vi "Write Signal Generator.lvclass.vi"(10 "Signal Generator.lvclass":refnum<class "Signal Generator.lvclass">, 11 "Harmonics in":refnum<class "Harmonics.lvclass">) -> (3 "Harmonics out":refnum<class "Harmonics.lvclass">)   [LabVIEW 2020, in "Harmonics.lvclass"]
uses:
  Harmonics.lvclass
  Instruments/Signal Generator/Signal Generator.lvclass
  Harmonics.lvclass/Harmonics.ctl
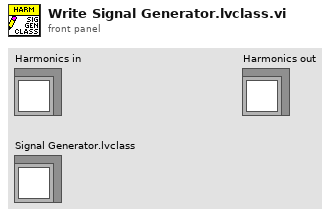
[diagram p1: front panel]
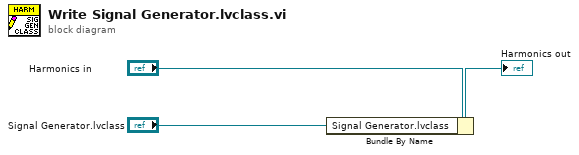
[diagram p0: block diagram]
diagram:
  n1 = Bundle By Name(cluster="Harmonics in", "Signal Generator.lvclass"="Signal Generator.lvclass") -> (→"Harmonics out":refnum<class "Harmonics.lvclass">)
